vi "Graph Data Insert.vi"(0 "Test Graph":refnum<vi>[](array[refnum])=[refnum, refnum, refnum, refnum, refnum, refnum, refnum, refnum, refnum, refnum], 1 "Item Name":string, 2 "Graph Index":i32, 3 "Loop Index":i32, 4 "Limit Data":cluster{"Frequency":dbl[], "Data In":dbl[]}[](array[cluster]), 5 "Data":T1, 6 "Pair Loop":i32, 7 "Pair Name":string, 9 "Graph Size":i32) -> ()   [LabVIEW 2011]
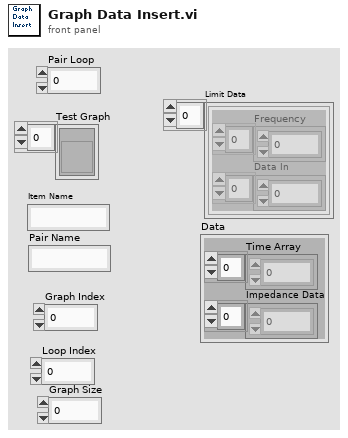
[diagram p1: front panel]
types:
  T1 = cluster{"Time Array":dbl[], "Impedance Data":dbl[]}
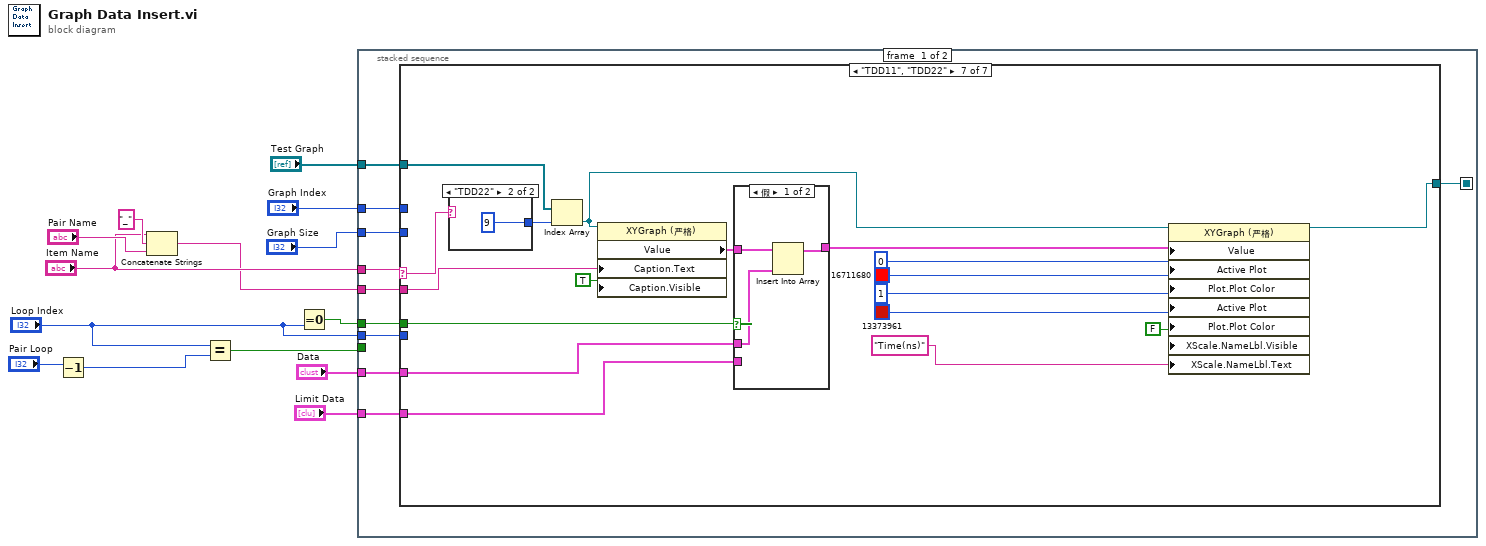
[diagram p0: block diagram]
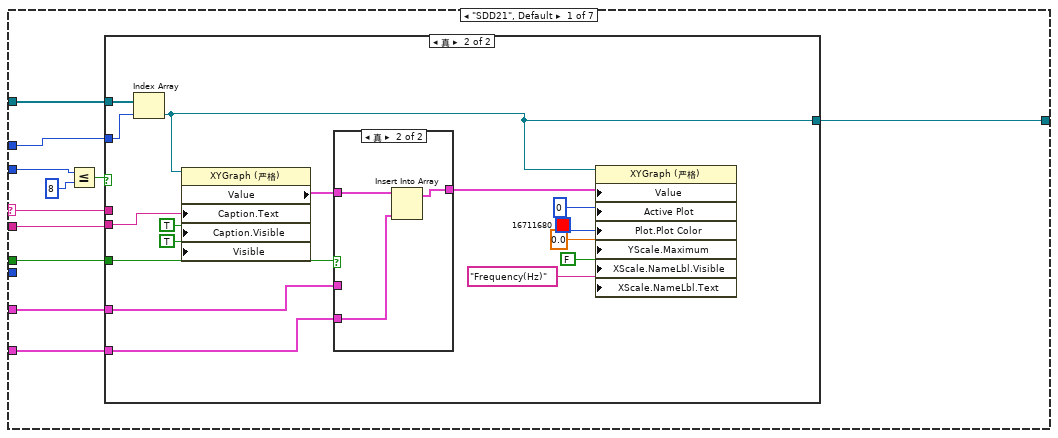
[diagram p2: hidden frame]
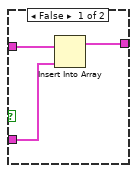
[diagram p4: hidden frame]
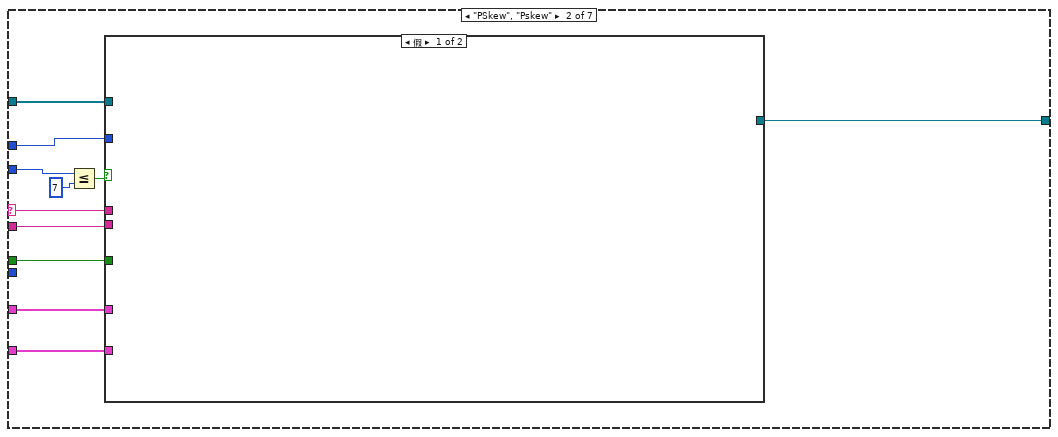
[diagram p5: hidden frame]
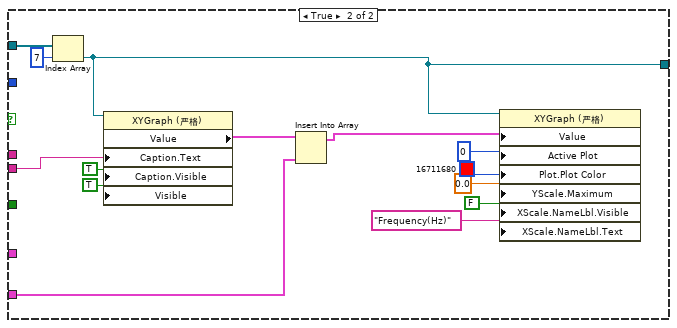
[diagram p6: hidden frame]
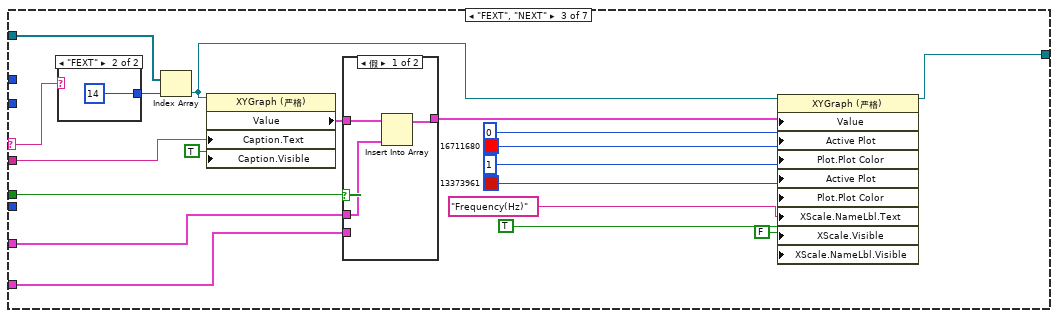
[diagram p7: hidden frame]
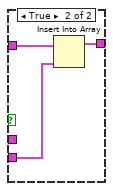
[diagram p8: hidden frame]
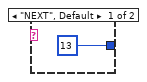
[diagram p9: hidden frame]
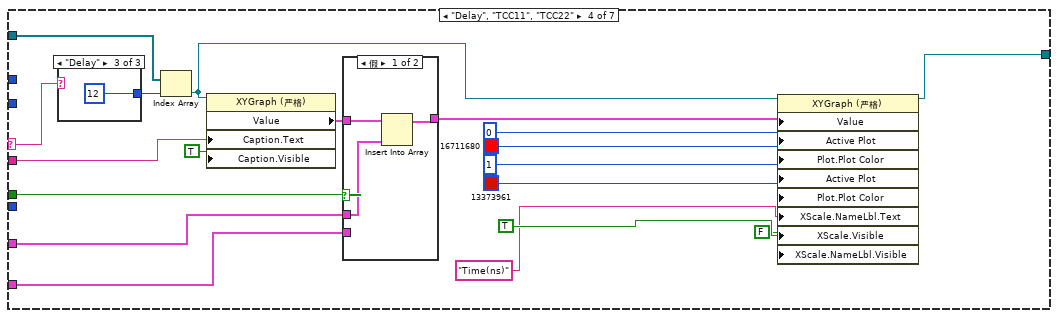
[diagram p10: hidden frame]
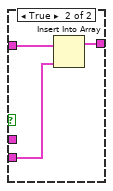
[diagram p11: hidden frame]
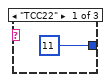
[diagram p12: hidden frame]
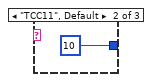
[diagram p13: hidden frame]
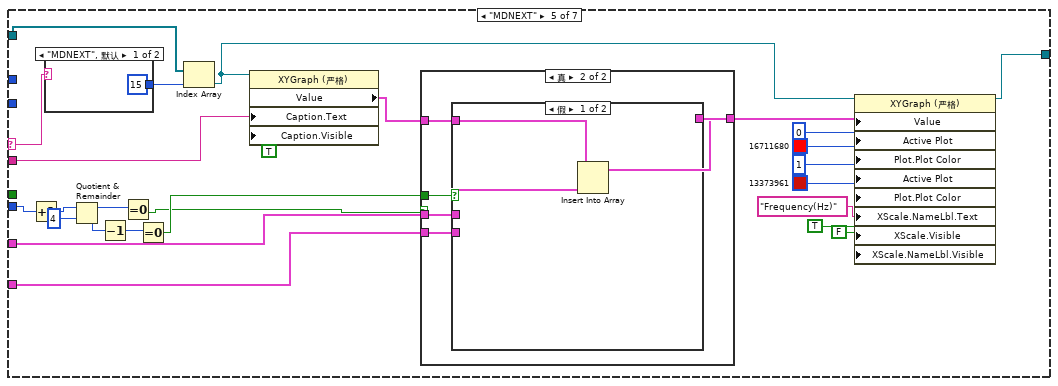
[diagram p14: hidden frame]
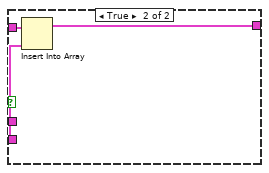
[diagram p16: hidden frame]
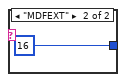
[diagram p17: hidden frame]
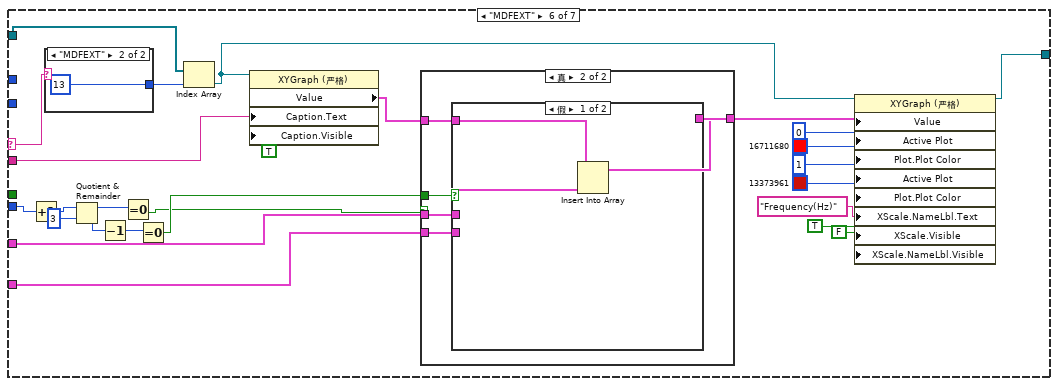
[diagram p18: hidden frame]
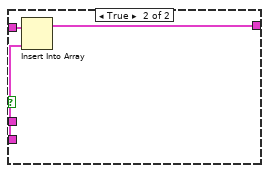
[diagram p20: hidden frame]
diagram:
  n1 = Decrement(x="Pair Loop") -> (x-1=w6:i32)
  n2 = Concatenate Strings("Item Name", "_" ("字符串"), "Pair Name") -> (w3:string)
  n3 = Equal?(x="Loop Index", y=w6) -> (x = y?=w4:bool)
  n4 = Equal To 0?(x="Loop Index") -> (x = 0?=w12:bool)
  n5 = stacked-sequence {
    seq-local: [w17 _] -> [_ w246]
    tunnel: "Graph Index" -> [w24 _]
    tunnel: "Test Graph" -> [w23 _]
    tunnel: w12 -> [w22 _]
    tunnel: "Data" -> [w21 _]
    tunnel: "Limit Data" -> [w20 _]
    tunnel: "Item Name" -> [w19 w244]
    tunnel: w3 -> [w18 _]
    tunnel: w4 -> [_ w245]
    tunnel: "Graph Size" -> [w16 _]
    tunnel: "Loop Index" -> [w15 _]
    frame #0 {
      n6 = case shown="\"TDD11\", \"TDD22\"" w19 {
        selector: w19 -> [w32 w65 w99 w126 w161 w201 w233]
        tunnel: w24 -> [w31 w64 _ _ _ _ _]
        tunnel: w23 -> [w33 w66 w100 w127 w162 w202 w234]
        tunnel: w22 -> [w30 w63 w98 w125 _ _ w232]
        tunnel: w21 -> [w29 w62 w96 w123 w159 w199 w230]
        tunnel: w20 -> [w28 w61 w95 w122 w158 w198 w229]
        tunnel: w18 -> [w27 w60 w87 w114 w150 w190 w221]
        tunnel: [w26 w59 w83 w111 w146 w186 w218] -> w17
        tunnel: w16 -> [w25 w58 _ _ _ _ _]
        tunnel: w15 -> [_ _ _ _ w145 w185 _]
        frame "SDD21", Default {
          n7 = Less Or Equal?(x=w25, y=8) -> (x <= y?=w34:bool)
          n8 = case shown="真" w34 {
            tunnel: w33 -> [_ w51]
            tunnel: w32 -> [_ _]
            tunnel: w31 -> [_ w50]
            tunnel: w30 -> [_ w49]
            tunnel: w29 -> [_ w46]
            tunnel: w28 -> [_ w47]
            tunnel: w27 -> [_ w40]
            tunnel: [_ w36] -> w26
            frame False {
            }
            frame True {
              n9 = Index Array(array=w51, index=w50) -> (element=w36:refnum<vi>)
              n10 = property class="XYGraph (严格)"(reference=w36, "Caption.Text"=w40, "Caption.Visible"=TRUE ("可见"), "Visible"=TRUE ("可见")) -> ("Value"=w48:cluster{"Horz Time array":dbl[], "Y":dbl[]}[])  [unwired: 1 in, 2 out]
              n11 = case shown="真" w49 {
                tunnel: w48 -> [w54 w57]
                tunnel: w47 -> [_ w56]
                tunnel: w46 -> [w53 _]
                tunnel: [w52 w55] -> w45
                frame False {
                  n12 = Insert Into Array(array=w54, new element=w53) -> (w52:cluster{"Horz Time array":dbl[], "Y":dbl[]}[])  [unwired: 1 in]
                }
                frame True {
                  n13 = Insert Into Array(array=w57, new element=w56) -> (w55:cluster{"Horz Time array":dbl[], "Y":dbl[]}[])  [unwired: 1 in]
                }
              }
              n14 = property class="XYGraph (严格)"(reference=w36, "Value"=w45, "Active Plot"=u32 0 ("活动曲线"), "Plot.Plot Color"=u32 16711680, "YScale.Maximum"=0.0 ("Y标尺.范围:最大值"), "XScale.NameLbl.Visible"=FALSE ("X标尺.名称标签.可见"), "XScale.NameLbl.Text"="Frequency(Hz)" ("X标尺.名称标签.文本")) -> ()  [unwired: 1 in, 2 out]
            }
          }
        }
        frame "PSkew", "Pskew" {
          n15 = Less Or Equal?(x=w58, y=7) -> (x <= y?=w67:bool)
          n16 = case shown="假" w67 {
            tunnel: w66 -> [_ w82]
            tunnel: w65 -> [_ _]
            tunnel: w64 -> [_ _]
            tunnel: w63 -> [_ _]
            tunnel: w62 -> [_ _]
            tunnel: w61 -> [_ w80]
            tunnel: w60 -> [_ w74]
            tunnel: [_ w70] -> w59
            frame False {
            }
            frame True {
              n17 = Index Array(array=w82, index=7 ("索引")) -> (element=w70:refnum<vi>)
              n18 = property class="XYGraph (严格)"(reference=w70, "Caption.Text"=w74, "Caption.Visible"=TRUE ("可见"), "Visible"=TRUE ("可见")) -> ("Value"=w81:cluster{"Horz Time array":dbl[], "Y":dbl[]}[])  [unwired: 1 in, 2 out]
              n19 = Insert Into Array(array=w81, new element=w80) -> (w79:cluster{"Horz Time array":dbl[], "Y":dbl[]}[])  [unwired: 1 in]
              n20 = property class="XYGraph (严格)"(reference=w70, "Value"=w79, "Active Plot"=u32 0 ("活动曲线"), "Plot.Plot Color"=u32 16711680, "YScale.Maximum"=0.0 ("Y标尺.范围:最大值"), "XScale.NameLbl.Visible"=FALSE ("X标尺.名称标签.可见"), "XScale.NameLbl.Text"="Frequency(Hz)" ("X标尺.名称标签.文本")) -> ()  [unwired: 1 in, 2 out]
            }
          }
        }
        frame "FEXT", "NEXT" {
          n21 = case shown="\"FEXT\"" w99 {
            tunnel: [13 ("Loop Index") 14 ("Loop Index")] -> w101
            frame "NEXT", Default {
            }
            frame "FEXT" {
            }
          }
          n22 = Index Array(array=w100, index=w101) -> (element=w94:refnum<vi>)
          n23 = property class="XYGraph (严格)"(reference=w94, "Caption.Text"=w87, "Caption.Visible"=TRUE ("标题.可见")) -> ("Value"=w97:cluster{"Horz Time array":dbl[], "Y":dbl[]}[])  [unwired: 1 in, 2 out]
          n24 = case shown="假" w98 {
            tunnel: w97 -> [w104 w107]
            tunnel: w96 -> [w103 _]
            tunnel: w95 -> [_ w106]
            tunnel: [w102 w105] -> w93
            frame False {
              n25 = Insert Into Array(array=w104, new element=w103) -> (w102:cluster{"Horz Time array":dbl[], "Y":dbl[]}[])  [unwired: 1 in]
            }
            frame True {
              n26 = Insert Into Array(array=w107, new element=w106) -> (w105:cluster{"Horz Time array":dbl[], "Y":dbl[]}[])  [unwired: 1 in]
            }
          }
          n27 = property class="XYGraph (严格)"(reference=w94, "Value"=w93, "Active Plot"=u32 0 ("活动曲线"), "Plot.Plot Color"=u32 16711680, "Active Plot"=u32 1 ("活动曲线"), "Plot.Plot Color"=u32 13373961, "XScale.NameLbl.Text"="Frequency(Hz)" ("X标尺.名称标签.文本"), "XScale.Visible"=TRUE ("X标尺.名称标签.可见"), "XScale.NameLbl.Visible"=FALSE ("X标尺.名称标签.可见")) -> (reference out=w83:refnum<vi>)  [unwired: 1 in, 1 out]
        }
        frame "Delay", "TCC11", "TCC22" {
          n28 = case shown="\"Delay\"" w126 {
            tunnel: [11 ("Loop Index") 10 ("Loop Index") 12 ("Loop Index")] -> w128
            frame "TCC22" {
            }
            frame "TCC11", Default {
            }
            frame "Delay" {
            }
          }
          n29 = Index Array(array=w127, index=w128) -> (element=w121:refnum<vi>)
          n30 = property class="XYGraph (严格)"(reference=w121, "Caption.Text"=w114, "Caption.Visible"=TRUE ("标题.可见")) -> ("Value"=w124:cluster{"Horz Time array":dbl[], "Y":dbl[]}[])  [unwired: 1 in, 2 out]
          n31 = case shown="假" w125 {
            tunnel: w124 -> [w131 w134]
            tunnel: w123 -> [w130 _]
            tunnel: w122 -> [_ w133]
            tunnel: [w129 w132] -> w120
            frame False {
              n32 = Insert Into Array(array=w131, new element=w130) -> (w129:cluster{"Horz Time array":dbl[], "Y":dbl[]}[])  [unwired: 1 in]
            }
            frame True {
              n33 = Insert Into Array(array=w134, new element=w133) -> (w132:cluster{"Horz Time array":dbl[], "Y":dbl[]}[])  [unwired: 1 in]
            }
          }
          n34 = property class="XYGraph (严格)"(reference=w121, "Value"=w120, "Active Plot"=u32 0 ("活动曲线"), "Plot.Plot Color"=u32 16711680, "Active Plot"=u32 1 ("活动曲线"), "Plot.Plot Color"=u32 13373961, "XScale.NameLbl.Text"="Time(ns)" ("X标尺.名称标签.文本"), "XScale.Visible"=TRUE ("X标尺.名称标签.可见"), "XScale.NameLbl.Visible"=FALSE ("X标尺.名称标签.可见")) -> (reference out=w111:refnum<vi>)  [unwired: 1 in, 1 out]
        }
        frame "MDNEXT" {
          n35 = Increment(x=w145) -> (x+1=w144:i32)
          n36 = case shown="\"MDNEXT\", 默认" w161 {
            tunnel: [15 ("Loop Index") 16 ("Loop Index")] -> w163
            frame "MDNEXT", Default {
            }
            frame "MDFEXT" {
            }
          }
          n37 = Quotient & Remainder(x=w144, y=4) -> (x-y*floor(x/y)=w142:i32, floor(x/y)=w141:i32)
          n38 = Decrement(x=w141) -> (x-1=w140:i32)
          n39 = Equal To 0?(x=w142) -> (x = 0?=w138:bool)
          n40 = Equal To 0?(x=w140) -> (x = 0?=w139:bool)
          n41 = Index Array(array=w162, index=w163) -> (element=w157:refnum<vi>)
          n42 = property class="XYGraph (严格)"(reference=w157, "Caption.Text"=w150, "Caption.Visible"=TRUE ("标题.可见")) -> ("Value"=w160:cluster{"Horz Time array":dbl[], "Y":dbl[]}[])  [unwired: 1 in, 2 out]
          n43 = case shown="真" w138 {
            tunnel: w160 -> [w164 w169]
            tunnel: w159 -> [_ w168]
            tunnel: w158 -> [_ w167]
            tunnel: [w164 w166] -> w156
            tunnel: w139 -> [_ w165]
            frame False {
            }
            frame True {
              n44 = case shown="假" w165 {
                tunnel: w169 -> [w172 w175]
                tunnel: w168 -> [w171 _]
                tunnel: w167 -> [_ w174]
                tunnel: [w170 w173] -> w166
                frame False {
                  n45 = Insert Into Array(array=w172, new element=w171) -> (w170:cluster{"Horz Time array":dbl[], "Y":dbl[]}[])  [unwired: 1 in]
                }
                frame True {
                  n46 = Insert Into Array(array=w175, new element=w174) -> (w173:cluster{"Horz Time array":dbl[], "Y":dbl[]}[])  [unwired: 1 in]
                }
              }
            }
          }
          n47 = property class="XYGraph (严格)"(reference=w157, "Value"=w156, "Active Plot"=u32 0 ("活动曲线"), "Plot.Plot Color"=u32 16711680, "Active Plot"=u32 1 ("活动曲线"), "Plot.Plot Color"=u32 13373961, "XScale.NameLbl.Text"="Frequency(Hz)" ("X标尺.名称标签.文本"), "XScale.Visible"=TRUE ("X标尺.名称标签.可见"), "XScale.NameLbl.Visible"=FALSE ("X标尺.名称标签.可见")) -> (reference out=w146:refnum<vi>)  [unwired: 1 in, 1 out]
        }
        frame "MDFEXT" {
          n48 = Increment(x=w185) -> (x+1=w184:i32)
          n49 = case shown="\"MDFEXT\"" w201 {
            tunnel: [15 ("Loop Index") 13 ("Loop Index")] -> w203
            frame "MDNEXT", Default {
            }
            frame "MDFEXT" {
            }
          }
          n50 = Quotient & Remainder(x=w184, y=3) -> (x-y*floor(x/y)=w182:i32, floor(x/y)=w181:i32)
          n51 = Decrement(x=w181) -> (x-1=w180:i32)
          n52 = Equal To 0?(x=w182) -> (x = 0?=w178:bool)
          n53 = Equal To 0?(x=w180) -> (x = 0?=w179:bool)
          n54 = Index Array(array=w202, index=w203) -> (element=w197:refnum<vi>)
          n55 = property class="XYGraph (严格)"(reference=w197, "Caption.Text"=w190, "Caption.Visible"=TRUE ("标题.可见")) -> ("Value"=w200:cluster{"Horz Time array":dbl[], "Y":dbl[]}[])  [unwired: 1 in, 2 out]
          n56 = case shown="真" w178 {
            tunnel: w200 -> [w204 w209]
            tunnel: w199 -> [_ w208]
            tunnel: w198 -> [_ w207]
            tunnel: [w204 w206] -> w196
            tunnel: w179 -> [_ w205]
            frame False {
            }
            frame True {
              n57 = case shown="假" w205 {
                tunnel: w209 -> [w212 w215]
                tunnel: w208 -> [w211 _]
                tunnel: w207 -> [_ w214]
                tunnel: [w210 w213] -> w206
                frame False {
                  n58 = Insert Into Array(array=w212, new element=w211) -> (w210:cluster{"Horz Time array":dbl[], "Y":dbl[]}[])  [unwired: 1 in]
                }
                frame True {
                  n59 = Insert Into Array(array=w215, new element=w214) -> (w213:cluster{"Horz Time array":dbl[], "Y":dbl[]}[])  [unwired: 1 in]
                }
              }
            }
          }
          n60 = property class="XYGraph (严格)"(reference=w197, "Value"=w196, "Active Plot"=u32 0 ("活动曲线"), "Plot.Plot Color"=u32 16711680, "Active Plot"=u32 1 ("活动曲线"), "Plot.Plot Color"=u32 13373961, "XScale.NameLbl.Text"="Frequency(Hz)" ("X标尺.名称标签.文本"), "XScale.Visible"=TRUE ("X标尺.名称标签.可见"), "XScale.NameLbl.Visible"=FALSE ("X标尺.名称标签.可见")) -> (reference out=w186:refnum<vi>)  [unwired: 1 in, 1 out]
        }
        frame "TDD11", "TDD22" {
          n61 = case shown="\"TDD22\"" w233 {
            tunnel: [8 ("Loop Index") 9 ("Loop Index")] -> w235
            frame "TDD11", Default {
            }
            frame "TDD22" {
            }
          }
          n62 = Index Array(array=w234, index=w235) -> (element=w228:refnum<vi>)
          n63 = property class="XYGraph (严格)"(reference=w228, "Caption.Text"=w221, "Caption.Visible"=TRUE ("标题.可见")) -> ("Value"=w231:cluster{"Horz Time array":dbl[], "Y":dbl[]}[])  [unwired: 1 in, 2 out]
          n64 = case shown="假" w232 {
            tunnel: w231 -> [w238 w241]
            tunnel: w230 -> [w237 _]
            tunnel: w229 -> [_ w240]
            tunnel: [w236 w239] -> w227
            frame False {
              n65 = Insert Into Array(array=w238, new element=w237) -> (w236:cluster{"Horz Time array":dbl[], "Y":dbl[]}[])  [unwired: 1 in]
            }
            frame True {
              n66 = Insert Into Array(array=w241, new element=w240) -> (w239:cluster{"Horz Time array":dbl[], "Y":dbl[]}[])  [unwired: 1 in]
            }
          }
          n67 = property class="XYGraph (严格)"(reference=w228, "Value"=w227, "Active Plot"=u32 0 ("活动曲线"), "Plot.Plot Color"=u32 16711680, "Active Plot"=u32 1 ("活动曲线"), "Plot.Plot Color"=u32 13373961, "XScale.NameLbl.Visible"=FALSE ("X标尺.名称标签.可见"), "XScale.NameLbl.Text"="Time(ns)" ("X标尺.名称标签.文本")) -> (reference out=w218:refnum<vi>)  [unwired: 1 in, 1 out]
        }
      }
    }
    frame #1 {
      n68 = case shown="假" w245 {
        tunnel: w246 -> [_ w248]
        tunnel: w244 -> [_ w247]
        frame False {
        }
        frame True {
          n69 = property class="XYGraph (严格)"(reference=w248, "Caption.Text"=w247) -> ()  [unwired: 1 in, 2 out]
        }
      }
    }
  }
